vi "FDV Meas Analyze FD Measurements.vi"(0 "Voltage Waveforms":waveform(dbl)[](array[waveform]), 11 "error in (no error)":errorcluster) -> (4 "Frequency Domain Measurements":T1 {"Detected Tones"."Amplitudes (V)" format="%.2p"; "Detected Tones"."Frequencies (Hz)" format="%.2p"}, 15 "error out":errorcluster)   [LabVIEW 2021, in "DAQ_Frequency Domain Measurement.lvlib"]
doc: "Analyzes the voltage waveforms data to derive required Frequency domain measurements"
uses:
  DAQ_Frequency Domain Measurement.lvlib
  Typedefs/FD Measurements.ctl
  Typedefs/Detected Tones.ctl
  <vilib>/Analysis/4window.llb/windowTd.ctl
  <vilib>/measure/maspectr.llb/FFT Spectrum (Mag-Phase) for N Chan.vi
  <vilib>/measure/matone.llb/Extract Multiple Tone Information 1 Chan.vi
  <vilib>/measure/NI_MAPro.lvlib
  <vilib>/Analysis/NI_AALPro.lvlib
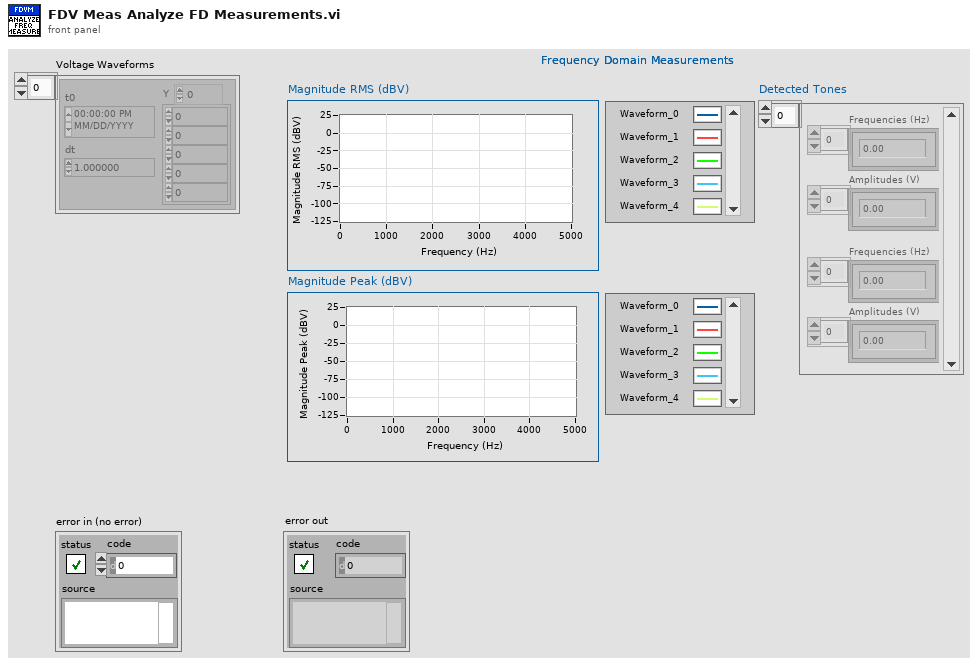
[diagram p1: front panel]
types:
  T1 = typedef "DAQ_Frequency Domain Measurement.lvlib/FD Measurements.ctl" = cluster{"Magnitude RMS (dBV)":cluster{"f0":dbl, "df":dbl, "magnitude":dbl[]}[], "Magnitude Peak (dBV)":cluster{"f0":dbl, "df":dbl, "magnitude":dbl[]}[], "Detected Tones":T2[]}
  T2 = typedef "DAQ_Frequency Domain Measurement.lvlib/Detected Tones.ctl" = cluster{"Frequencies (Hz)":dbl[], "Amplitudes (V)":dbl[]}
  T3 = enum32{"none", "input signal", "detected signal", "residual signal"}
  T4 = typedef "NI_AALPro.lvlib/windowTd.ctl" = u32
  T5 = cluster{"averaging mode":enum16{"No averaging", "Vector averaging", "RMS averaging", "Peak hold"}, "weighting mode":enum16{"Linear", "Exponential"}, "number of averages":u32}
  T6 = cluster{"dB On (F)":bool, "unwrap phase (F)":bool, "convert to degree (F)":bool}
  T7 = cluster{"detected frequency":dbl, "detected amplitude":dbl, "detected phase (deg)":dbl}[]
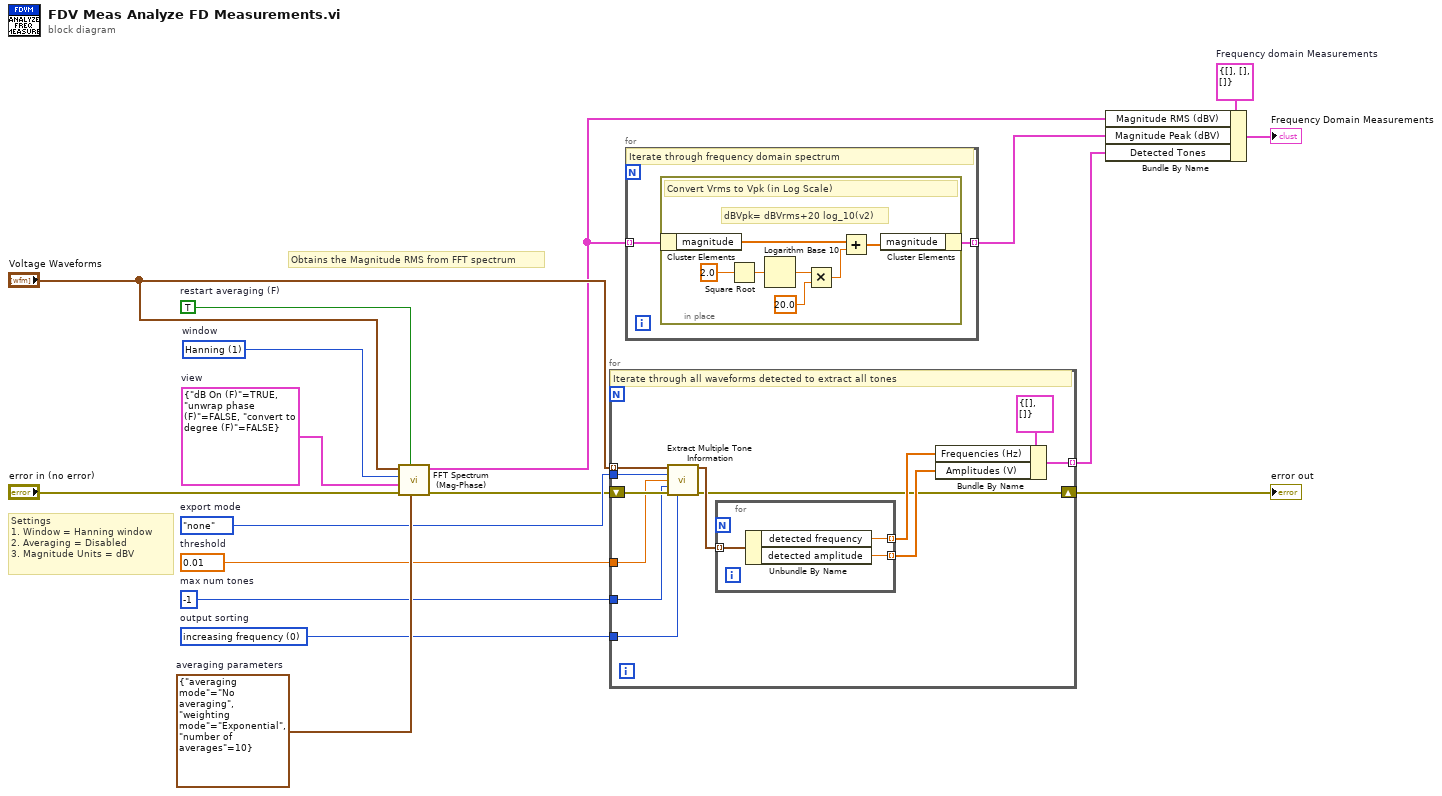
[diagram p0: block diagram]
diagram:
  w1 = -1  # max num tones
  w2 = 0.01  # threshold
  w4 = 0 items=["increasing frequency", "decreasing amplitude"]  # output sorting
  w9 = T3."none"  # export mode
  w14 = T4 1 items=["Rectangle"=0, "Hanning"=1, "Hamming"=2, "Blackman-Harris"=3, "Exact Blackman"=4, "Blackman"=5, "Flat Top"=6, "4 Term B-Harris "=7, "7 Term B-Harris"=8, "Low Sidelobe"=9, "Blackman Nuttall"=11, "Triangle"=30, "Bartlett-Hanning"=31, "Bohman"=32, "Parzen"=33, "Welch"=34, "Kaiser"=60, "Dolph-Chebyshev"=61, "Gaussian"=62]  # window
  w12 = T5 {"averaging mode"=enum."No averaging", "weighting mode"=enum."Exponential", "number of averages"=10}  # averaging parameters
  w13 = T6 {"dB On (F)"=TRUE, "unwrap phase (F)"=FALSE, "convert to degree (F)"=FALSE}  # view
  w15 = TRUE  # restart averaging (F)
  w17 = T1 {"Magnitude RMS (dBV)"=[], "Magnitude Peak (dBV)"=[], "Detected Tones"=[]}  # Frequency domain Measurements
  # "Settings\n1. Window = Hanning window\n2. Averaging = Disabled\n3. Magnitude Units = dBV"
  # "Obtains the Magnitude RMS from FFT spectrum"
  n1 = call-poly <vilib>:"FFT Spectrum (Mag-Phase).vi"("averaging parameters"=w12, "restart averaging (F)"=w15, "error in (no error)"="error in (no error)", "view"=w13, "window"=w14, "time signals"="Voltage Waveforms") -> ("error out"=w8:errorcluster, "magnitudes"=w6:cluster{"f0":dbl, "df":dbl, "magnitude":dbl[]}[])  [unwired: 1 in, 3 out]
  n2 = for {
    tunnel: "Voltage Waveforms" -> [w21] mode=indexing
    tunnel: w9 -> [w29]
    shift-right: [w20] -> w7
    shift-left: w8 -> [w28]
    tunnel: w4 -> [w27]
    tunnel: [w22] -> w3 mode=indexing
    tunnel: w2 -> [w19]
    tunnel: w1 -> [w18]
    # "Iterate through all waveforms detected to extract all tones"
    n3 = call-poly <vilib>:"Extract Multiple Tone Information.vi"("time signal in"=w21, "export mode"=w29, "threshold"=w19, "max num tones"=w18, "error in (no error)"=w28, "output sorting"=w27) -> ("multiple tone information"=w25:T7, "error out"=w20:errorcluster)  [unwired: 7 in, 1 out]
    n4 = for {
      tunnel: w25 -> [w32] mode=indexing
      tunnel: [w31] -> w24 mode=indexing
      tunnel: [w30] -> w23 mode=indexing
      n5 = Unbundle By Name(w32) -> ("detected frequency"=w31:dbl, "detected amplitude"=w30:dbl)
    }
    n6 = Bundle By Name(cluster=T2 {"Frequencies (Hz)"=[], "Amplitudes (V)"=[]} ("Detected Tone"), "Frequencies (Hz)"=w24, "Amplitudes (V)"=w23) -> (w22:T2)
  }
  "error out" <- w7
  n7 = for {
    tunnel: w6 -> [w34] mode=indexing
    tunnel: [w33] -> w5 mode=indexing
    # "Iterate through frequency domain spectrum"
    n8 = in-place {
      # "dBVpk= dBVrms+20 log_10(v2)"
      # "Convert Vrms to Vpk (in Log Scale)"
      n9 = in-place-cluster #1(w34) -> ("magnitude"=w41:dbl[])
      n10 = Square Root(x=2.0) -> (sqrt(x)=w35:dbl)
      n11 = Logarithm Base 10(1:w35) -> (0:w38:dbl)
      n12 = Multiply(x=w38, y=20.0) -> (x*y=w36:dbl)
      n13 = Add(x=w41, y=w36) -> (x+y=w39:dbl[])
      n14 = in-place-cluster #1("magnitude"=w39) -> (w33:cluster{"f0":dbl, "df":dbl, "magnitude":dbl[]})
    }
  }
  n15 = Bundle By Name(cluster=w17, "Magnitude RMS (dBV)"=w6, "Magnitude Peak (dBV)"=w5, "Detected Tones"=w3) -> (→"Frequency Domain Measurements":T1)
